vi "Motor_Encoder_UART_Kadjst.vi"() -> ()   [LabVIEW 2025]
uses:
  <vilib>/Instr/_visa.llb/VISA Configure Serial Port (Instr).vi
panel:
  out "Error Chart":i32(graph)
  in  "Ki":dbl(knob) scale=0.0..0.01
  in  "Kd":dbl(knob) scale=0.0..0.01
  in  "Kp":dbl(knob) scale=0.0..1.0
  in  "VISA resource name":refnum<visa-resource-name>
  out "error out":errorcluster
  in  "write":bool
  in  "buffer size":u32=256
  in  "timeout (ms)":u32=10000
  in  "flow control":u16
  in  "stop bits":u16=10
  in  "parity":u16(ring) items=["None", "Odd", "Even", "Mark", "Space"]
  in  "data bits":u16=8 min=5 max=8 step=1
  in  "baud rate":u32=9600
  out "read string":string
  in  "Set-Point":string
  in  "stop":bool
  # "Control motor - encoder Arduino UNO"
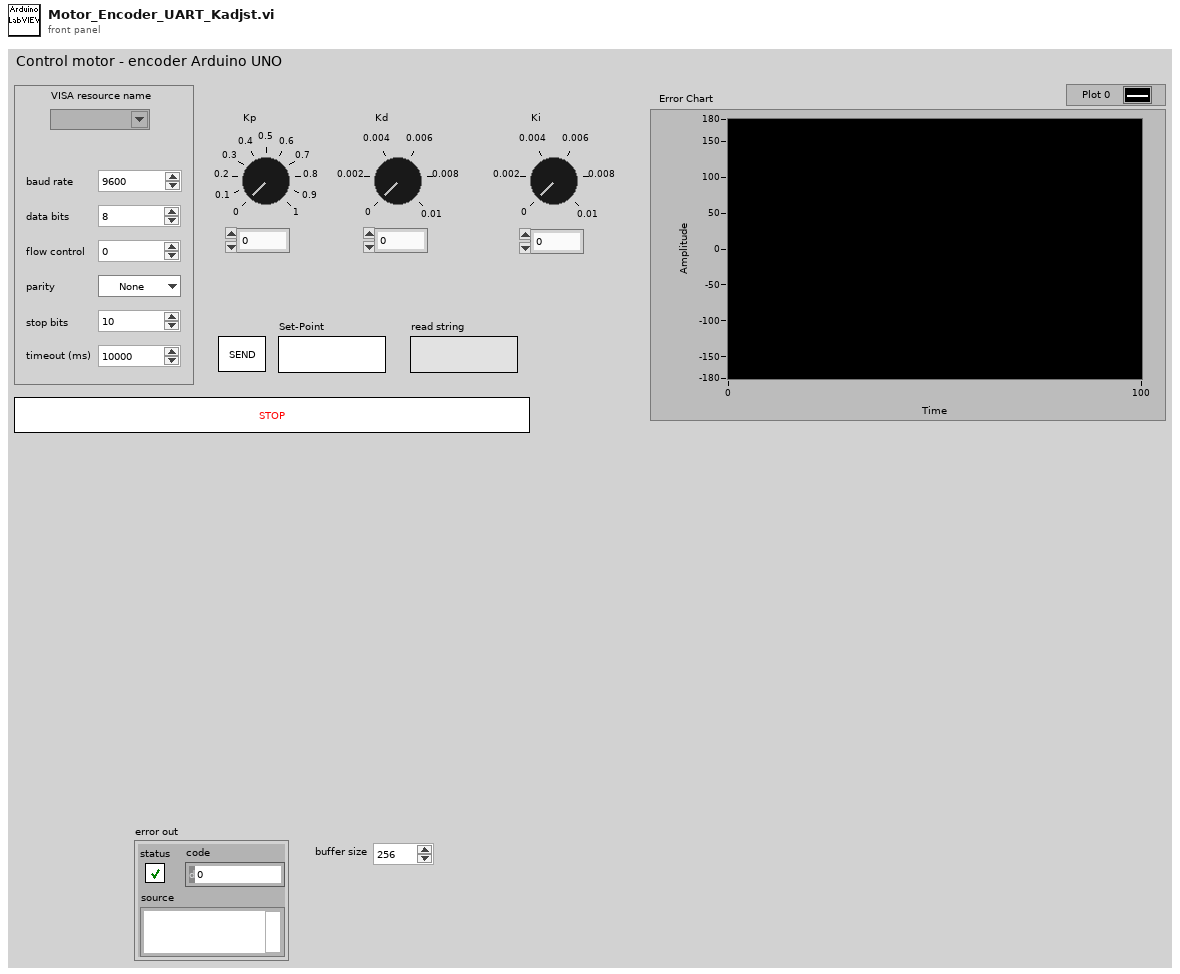
[diagram p1: front panel]
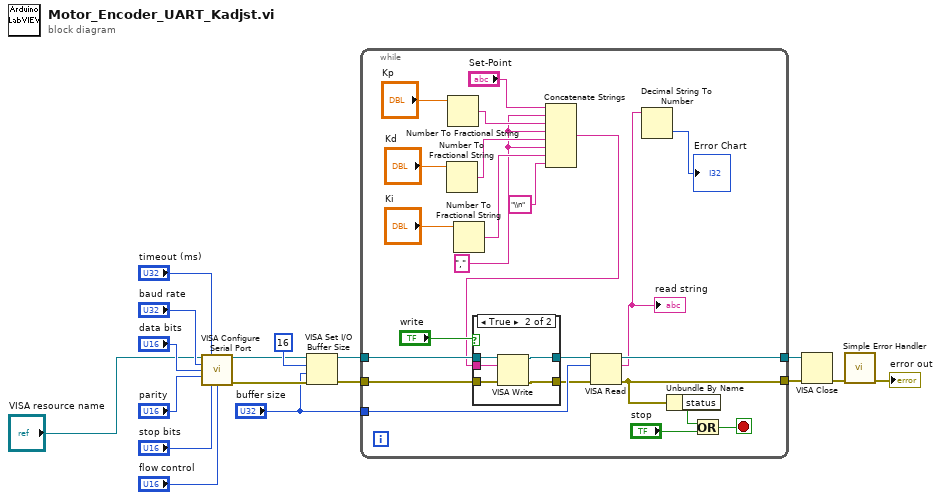
[diagram p0: block diagram]
diagram:
  n1 = call-poly "VISA Configure Serial Port"("VISA resource name"="VISA resource name", "timeout (10sec)"="timeout (ms)", "baud rate (9600)"="baud rate", "data bits (8)"="data bits", "parity (0:none)"="parity", "stop bits (10: 1 bit)"="stop bits", "flow control (0:none)"="flow control") -> ("VISA resource name out"=w8:refnum<visa-resource-name>, "error out"=w7:errorcluster)  [unwired: 7 in]
  n2 = VISA Set I/O Buffer Size(VISA resource name=w8, mask (16)=u16 16 ("I/O Receive\nBuffer mask"), size (4096)="buffer size", error in (no error)=w7) -> (VISA resource name out=w6:refnum<visa-resource-name>, error out=w5:errorcluster)
  n3 = while {
    tunnel: w6 -> [w34]
    tunnel: w5 -> [w33]
    tunnel: [w35] -> w17
    tunnel: [w37] -> w16
    tunnel: "buffer size" -> [w36]
    stop <- w38 stop-if-true
    w20 = "," ("string")
    n4 = Number To Fractional String(number="Kd") -> (F-format string=w23:string)  [unwired: 3 in]
    n5 = Number To Fractional String(number="Kp") -> (F-format string=w24:string)  [unwired: 3 in]
    n6 = Number To Fractional String(number="Ki") -> (F-format string=w22:string)  [unwired: 3 in]
    n7 = Concatenate Strings("Set-Point", w20, w24, w20, w23, w20, w22, "\\n" ("string")) -> (w26:string)
    n8 = case shown="True" "write" {
      tunnel: w34 -> [w42 w47]
      tunnel: w33 -> [w41 w46]
      tunnel: [w42 w45] -> w32
      tunnel: [w41 w44] -> w31
      tunnel: w26 -> [_ w43]
      frame False {
      }
      frame True {
        n9 = VISA Write(VISA resource name=w47, write buffer=w43, error in (no error)=w46) -> (VISA resource name out=w45:refnum<visa-resource-name>, error out=w44:errorcluster)  [unwired: 1 out]
      }
    }
    n10 = VISA Read(VISA resource name=w32, byte count=w36, error in (no error)=w31) -> (VISA resource name out=w35:refnum<visa-resource-name>, read buffer=w19:string, error out=w37:errorcluster)  [unwired: 1 out]
    "read string" <- w19
    n11 = Decimal String To Number(string=w19) -> (number=→"Error Chart":i32)  [unwired: 2 in, 1 out]
    n12 = Unbundle By Name(w37) -> ("status"=w40:bool)
    n13 = Or(x=w40, y="stop") -> (x .or. y?=w38:bool)
  }
  n14 = VISA Close(VISA resource name=w17, error in (no error)=w16) -> (error out=w3:errorcluster)
  n15 = call <vilib>:"Simple Error Handler.vi"("error in (no error)"=w3) -> ("error out"=→"error out":errorcluster)  [unwired: 4 in, 4 out]
